vi "Ejercicio 2.4.vi"() -> ()   [LabVIEW 2020]
panel:
  out "Resultado:":string
  out "Resultado:":string
  out "Resultado:":string
  out "Resultado:":string
  in  "Numero 2":dbl
  in  "Número 1":dbl
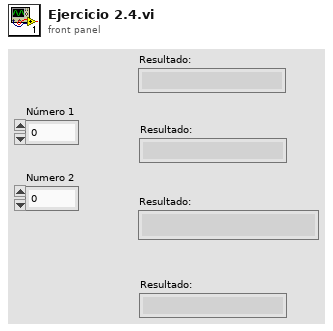
[diagram p1: front panel]
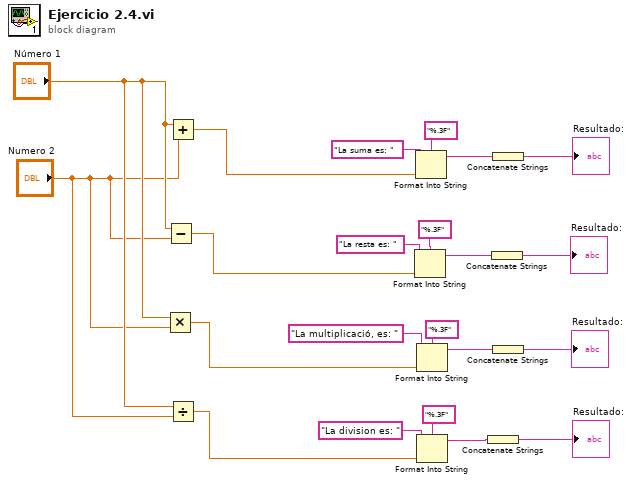
[diagram p0: block diagram]
diagram:
  n1 = Multiply(x="Número 1", y="Numero 2") -> (x*y=w3:dbl)
  n2 = Subtract(x="Número 1", y="Numero 2") -> (x-y=w2:dbl)
  n3 = Add(x="Número 1", y="Numero 2") -> (x+y=w1:dbl)
  n4 = Divide(x="Número 1", y="Numero 2") -> (x/y=w19:dbl)
  n5 = Format Into String(format string="%.3F", initial string="La resta es: ", w2) -> (resulting string=w9:string)  [unwired: 1 in, 1 out]
  n6 = Format Into String(format string="%.3F", initial string="La suma es: ", w1) -> (resulting string=w6:string)  [unwired: 1 in, 1 out]
  n7 = Format Into String(format string="%.3F", initial string="La multiplicació, es: ", w3) -> (resulting string=w14:string)  [unwired: 1 in, 1 out]
  n8 = Format Into String(format string="%.3F", initial string="La division es: ", w19) -> (resulting string=w17:string)  [unwired: 1 in, 1 out]
  n9 = Concatenate Strings(w17) -> (→"Resultado:":string)
  n10 = Concatenate Strings(w9) -> (→"Resultado:":string)
  n11 = Concatenate Strings(w6) -> (→"Resultado:":string)
  n12 = Concatenate Strings(w14) -> (→"Resultado:":string)
